vi "Create.vi"(10 "APIs":refnum<class "API.lvclass">[](array[class])) -> (3 "ApiArrayValue out":refnum<class "ApiArrayValue.lvclass">)   [LabVIEW 2020, in "Volatus.lvlib" / "ApiArrayValue.lvclass"]
uses:
  ApiArrayValue.lvclass
  ApiArrayValue.lvclass/ApiArrayValue.ctl
  API/API.lvclass
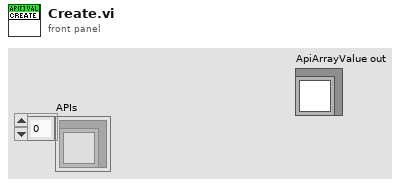
[diagram p1: front panel]
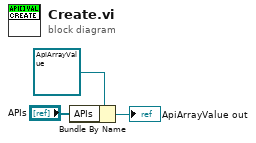
[diagram p0: block diagram]
diagram:
  n1 = Bundle By Name(cluster=refnum<class "ApiArrayValue.lvclass"> refnum ("ApiArrayValue in"), "APIs"="APIs") -> (→"ApiArrayValue out":refnum<class "ApiArrayValue.lvclass">)
